vi "Set Panel State.vi"(10 "Front Panel Window:State":T1(ring)) -> (2 "Msg Strategy":refnum<class "Msg Strategy.lvclass">)   [LabVIEW 2021, in "Set Panel State Msg Strategy.lvlib"]
uses:
  Set Panel State Msg Strategy.lvlib
  jettl/Msg Strategy/Msg Strategy.lvclass
  Set Panel State Msg Strategy/Set Panel State Msg Strategy.lvclass
  C:/git/jettl/jettl/jettl/Msg Strategy/Msg Strategy.lvclass
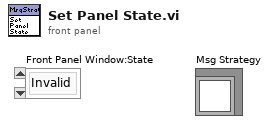
[diagram p1: front panel]
types:
  T1 = enum32{"Invalid", "Standard", "Closed", "Hidden", "Minimized", "Maximized"}
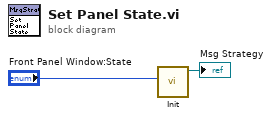
[diagram p0: block diagram]
diagram:
  n1 = call "Init.vi"("Front Panel Window:State"="Front Panel Window:State") -> ("Set Panel State Msg Strategy out"=→"Msg Strategy":refnum<class "Set Panel State Msg Strategy.lvclass">)  [unwired: 10 in]
